vi "Set VI Description and Help.vi"(4 "Help Tag":string, 6 "Help Path":string, 9 "VI Description":string, 10 "VI Index":i32, 11 "VI Data in":T1[](array[typedef])) -> (3 "VI Data out":T1[](array[typedef]))   [LabVIEW 2023, in "VI Properties Editor.lvlib"]
uses:
  VI Properties Editor.lvlib
  CTLs/VI Data.ctl
  <vilib>/picture/picture.llb/imagedata.ctl
  CTLs/VI Properties.ctl
  CTLs/Control Properties.ctl
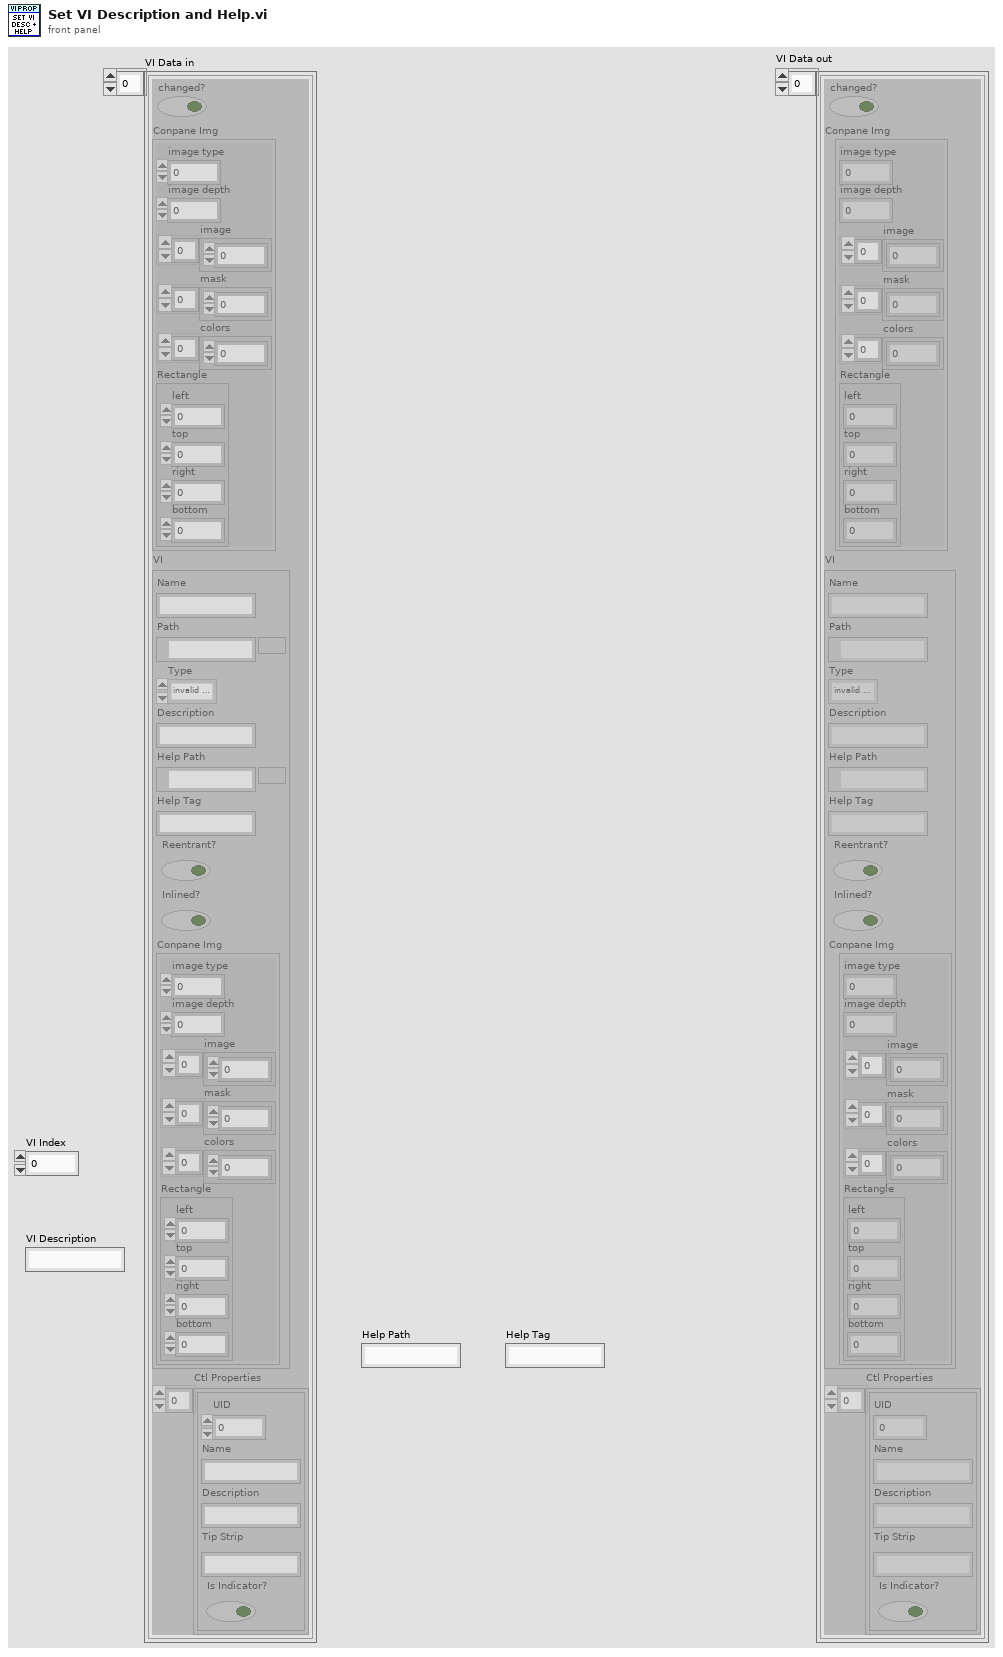
[diagram p1: front panel]
types:
  T1 = typedef "VI Properties Editor.lvlib/VI Data.ctl" = cluster{"changed?":bool, "Conpane Img":T2, "VI":T3, "Ctl Properties":T4[]}
  T2 = typedef "imagedata.ctl" = cluster{"image type":i32, "image depth":i32, "image":u8[], "mask":u8[], "colors":u32[], "Rectangle":cluster{"left":i16, "top":i16, "right":i16, "bottom":i16}}
  T3 = typedef "VI Properties Editor.lvlib/VI Properties.ctl" = cluster{"Name":string, "Path":path, "Type":enum32{"invalid VI type", "Standard VI", "Control VI", "Global VI", "Polymorphic VI", "Configuration VI", "SubSystem", "Facade VI", "Method VI", "Statechart Diagram VI"}, "Description":string, "Help Path":path, "Help Tag":string, "Reentrant?":bool, "Inlined?":bool, "Conpane Img":T2}
  T4 = typedef "VI Properties Editor.lvlib/Control Properties.ctl" = cluster{"UID":i32, "Name":string, "Description":string, "Tip Strip":string, "Is Indicator?":bool}
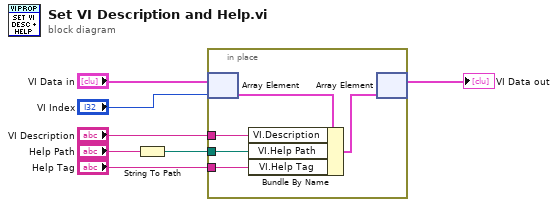
[diagram p0: block diagram]
diagram:
  n1 = String To Path(string="Help Path") -> (path=w1:path)
  n2 = in-place {
    in-place-border: "VI Description" -> [w11]
    in-place-border: w1 -> [w10]
    in-place-border: "Help Tag" -> [w9]
    n3 = in-place-array #1("VI Data in", "VI Index") -> (w12:T1)
    n4 = Bundle By Name(cluster=w12, "VI.Description"=w11, "VI.Help Path"=w10, "VI.Help Tag"=w9) -> (w8:T1)
    n5 = in-place-array #1(w8) -> (→"VI Data out":T1[])  [unwired: 1 out]
  }
